vi "Script Checker.vi"(8 "error in (no error)":errorcluster, 10 "Run":refnum<class "Run Instance.lvclass">, 11 "Monkey in":refnum<class "Monkey.lvclass">) -> (0 "error out":errorcluster, 1 "Correct Build?":bool, 2 "Script exists?":bool, 3 "Monkey out":refnum<class "Monkey.lvclass">)   [LabVIEW 2020, in "Monkey.lvlib" / "Monkey.lvclass"]
doc: "This VI checks if the script to be run on Sinara exists (taking into account the value of Dummy?), and in case it saves it into the class private data."
uses:
  Monkey.lvclass
  Run Utilities/Run Instance/Run Instance.lvclass
  Ancestor/Ancestor/Ancestor.lvclass/Ancestor.ctl
  FGV/Error Memory/Get Error Description.vi
  Support VIs/Get PC name.vi
  Ancestor/Ancestor/Read ID.vi
  Support VIs/Get Class Name.vi
  <vilib>/Utility/error.llb/Clear Errors.vi
  FGV/Error Memory/Error Memory Core.vi
  <vilib>/AdvancedString/Delimited String to 1D String Array.vi
  Support VIs/Circus Root Path.vi
  FGV/Error Memory/Error Crt Lvl checker.vi
  FGV/Error Memory/Error Memory Core.vi/40c8088d-b597-4017-91af-faa98e00292e.vi
  FGV/Error Memory/Error Memory Core.vi/d4a3ab98-063c-4e44-b43d-fbdcfe6c2be2.vi
  Support VIs/Global Memory.vi
  <vilib>/Utility/LVClass/Get LV Class Name.vi
  Support VIs/Is in Packed Library.vi
  Support VIs/TALOS Root path.vi
  Support VIs/Read CSV worksheet.vi
  Support VIs/Global Constants.vi
  <vilib>/Utility/error.llb/General Error Handler.vi
  Ancestor/Ancestor/Ancestor.lvclass
  <vilib>/Comparison/Equal/Equal Functor/Equal Functor.lvclass
  Interfaces/FPGA Interface/FPGA Interface.lvclass
  TALOS.lvlib
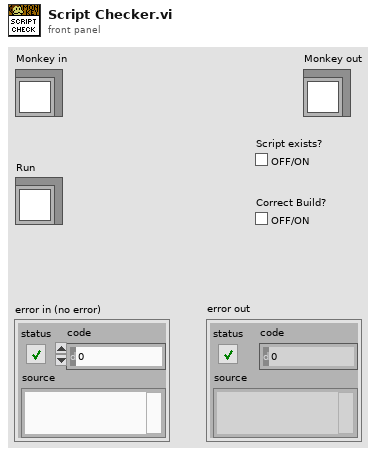
[diagram p1: front panel]
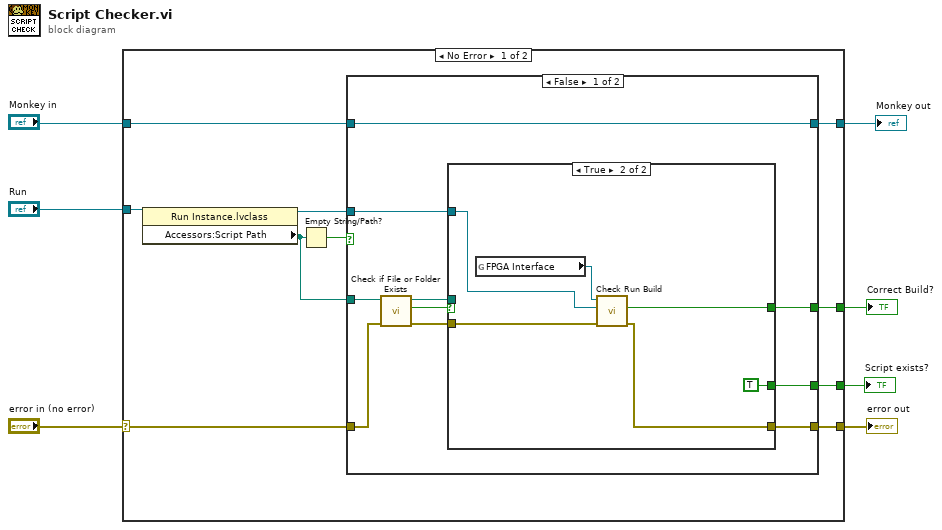
[diagram p0: block diagram]
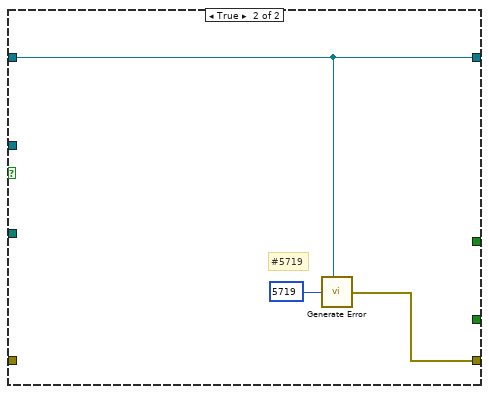
[diagram p3: hidden frame]
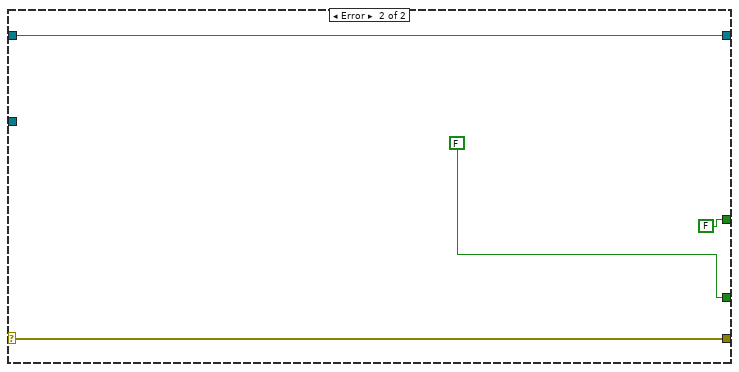
[diagram p4: hidden frame]
diagram:
  n1 = case shown="No Error" "error in (no error)" {
    selector: "error in (no error)" -> [w12 w40]
    tunnel: [w17 w40] -> w7
    tunnel: [w15 w39] -> w6
    tunnel: "Monkey in" -> [w14 w39]
    tunnel: [w13 FALSE ("file or folder exists?")] -> w4
    tunnel: "Run" -> [w10 _]
    tunnel: [w11 FALSE] -> w2
    frame No Error {
      n2 = property class="Run Instance.lvclass"(reference=w10) -> (reference out=w8:refnum<class "Run Instance.lvclass">, "Accessors:Script Path"=w9:path)  [unwired: 1 in, 1 out]
      n3 = Empty String/Path?(string/path=w9) -> (empty?=w16:bool)
      n4 = case shown="False" w16 {
        tunnel: [w18 w35] -> w15
        tunnel: w14 -> [w18 w35]
        tunnel: w12 -> [w27 _]
        tunnel: [w22 w37] -> w17
        tunnel: [w23 _] -> w13
        tunnel: w9 -> [w26 _]
        tunnel: [w20 _] -> w11
        tunnel: w8 -> [w19 _]
        frame False {
          n5 = call <vilib>:"Check if File or Folder Exists.vi"("error in (no error)"=w27, "path"=w26) -> ("error out"=w24:errorcluster, "file or folder exists?"=w25:bool, "dup path"=w21:path)  [unwired: 7 in]
          n6 = case shown="True" w25 {
            tunnel: w24 -> [w28 w34]
            tunnel: [_ TRUE] -> w23
            tunnel: [w28 w32] -> w22
            tunnel: w21 -> [_ _]
            tunnel: [_ w33] -> w20
            tunnel: w19 -> [_ w30]
            frame False {
            }
            frame True {
              n7 = global read "Global Memory.vi" "FPGA Interface"() -> (w29:refnum<class "FPGA Interface.lvclass">)
              n8 = call-dynamic "Check Run Build.vi"("error in (no error)"=w34, "Run"=w30, "FPGA Interface in"=w29) -> ("error out"=w32:errorcluster, "Correct Build"=w33:bool)  [unwired: 7 in]
            }
          }
        }
        frame True {
          # "#5719"
          n9 = call "Generate Error.vi"("Class"=w35, "Error Code"=5719) -> ("error out"=w37:errorcluster)  [unwired: 5 in]
        }
      }
    }
    frame Error {
    }
  }
  "error out" <- w7
  "Monkey out" <- w6
  "Script exists?" <- w4
  "Correct Build?" <- w2
